vi "Read Attributes.vi"(11 "Blackstart Microgrid Msg":refnum<class "Blackstart Microgrid Msg.lvclass">) -> (2 "Payload":cluster{"Data":variant})   [LabVIEW 2018, in "Remote Operation Abstract.lvlib" / "Blackstart Microgrid Msg.lvclass"]
uses:
  Blackstart Microgrid Msg.lvclass
  Blackstart Microgrid Msg.lvclass/Blackstart Microgrid Msg.ctl
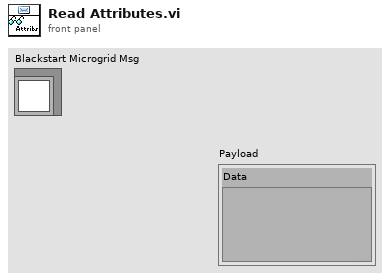
[diagram p1: front panel]
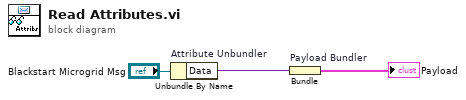
[diagram p0: block diagram]
diagram:
  n1 = Unbundle By Name "Attribute Unbundler"("Blackstart Microgrid Msg") -> ("Data"=w1:variant)
  n2 = Bundle "Payload Bundler"("Data"=w1) -> (→"Payload":cluster{"Data":variant})  [unwired: 1 in]
